vi "LSCI 370 Data Analog Output.vi"(0 "VISA session":refnum<visa-resource-name>, 5 "Analog Channel (0: Analog Out 1)":u16(ring) items=["Analog Out 1", "Analog Out 2"], 11 "error in (no error)":errorcluster) -> (4 "dup VISA session":refnum<visa-resource-name>, 8 "Analog Output":dbl min=-100.0 max=100.0 step=1e-05 format="%^.5e", 15 "error out":errorcluster)   [LabVIEW 2018]
doc: "This VI querys the instrument for the percentage of output of the analog output."
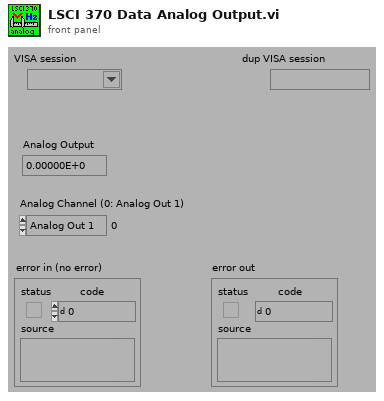
[diagram p1: front panel]
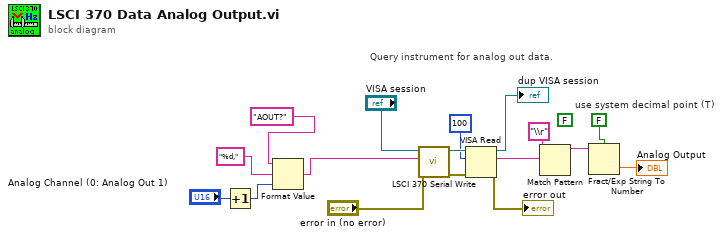
[diagram p0: block diagram]
diagram:
  (unwired) FALSE ("use system decimal point (T)")
  w7 = FALSE  # use system decimal point (T)
  # "Query instrument for analog out data."
  n1 = Increment(x="Analog Channel (0: Analog Out 1)") -> (x+1=w2:u16)
  n2 = Format Value(string ("")="AOUT?", format string="%d,", value (0)=w2) -> (output string=w1:string)
  n3 = call "LSCI 370 Serial Write.vi"("error in (no error)"="error in (no error)", "Write Buffer (\"\")"=w1, "VISA session"="VISA session") -> ("error out"=w16:errorcluster, "dup VISA session"=w17:refnum<visa-resource-name>)  [unwired: 6 in, 1 out]
  n4 = VISA Read(VISA resource name=w17, byte count=100, error in (no error)=w16) -> (VISA resource name out=→"dup VISA session":refnum<visa-resource-name>, read buffer=w14:string, error out=→"error out":errorcluster)  [unwired: 1 out]
  n5 = Match Pattern(string=w14, regular expression="\\r") -> (before substring=w12:string)  [unwired: 1 in, 3 out]
  n6 = Fract/Exp String To Number(use system decimal point (T)=w7, string=w12) -> (number=→"Analog Output":dbl)  [unwired: 2 in, 1 out]
